vi "Get Directions.vi"(11 "Proto in":refnum<class "Numeric Keypad.lvclass">) -> (2 "Directional Button Presses":string[](array[string]), 3 "Proto out":refnum<class "Numeric Keypad.lvclass">)   [LabVIEW 2020, in "Numeric Keypad.lvclass"]
uses:
  Numeric Keypad.lvclass
  Numeric Keypad.lvclass/Numeric Keypad.ctl
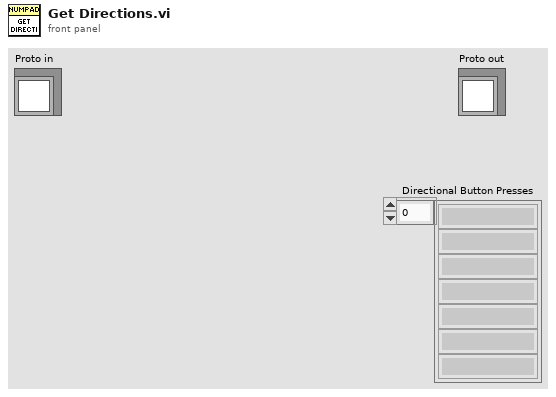
[diagram p1: front panel]
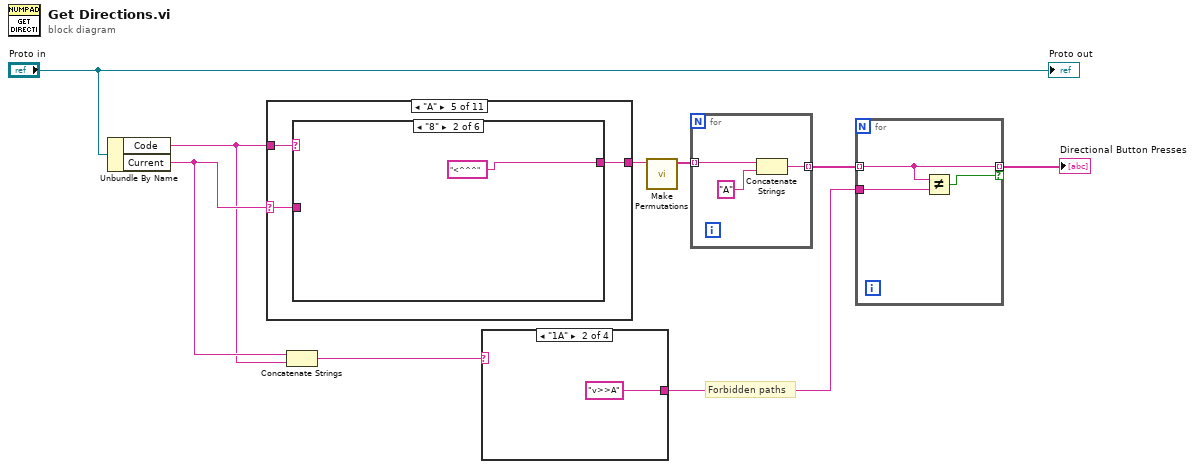
[diagram p0: block diagram]
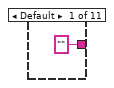
[diagram p2: hidden frame]
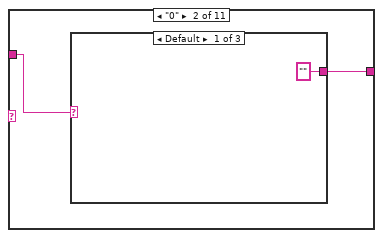
[diagram p3: hidden frame]
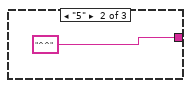
[diagram p4: hidden frame]
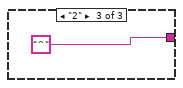
[diagram p5: hidden frame]
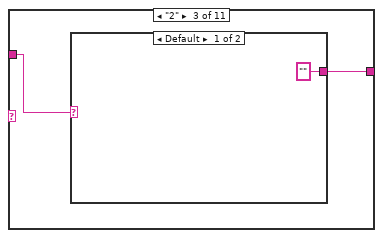
[diagram p6: hidden frame]
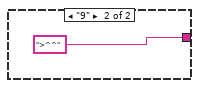
[diagram p7: hidden frame]
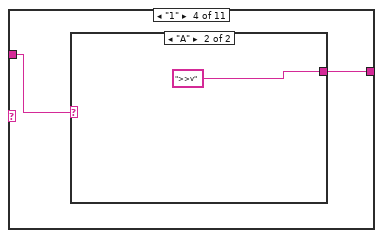
[diagram p8: hidden frame]
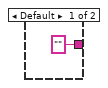
[diagram p9: hidden frame]
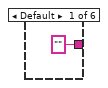
[diagram p10: hidden frame]
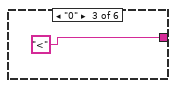
[diagram p11: hidden frame]
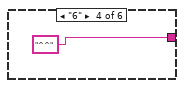
[diagram p12: hidden frame]
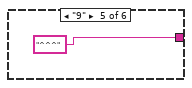
[diagram p13: hidden frame]
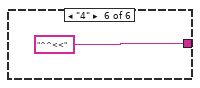
[diagram p14: hidden frame]
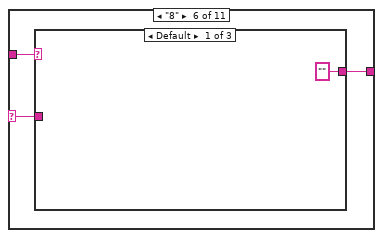
[diagram p15: hidden frame]
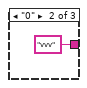
[diagram p16: hidden frame]
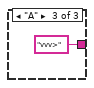
[diagram p17: hidden frame]
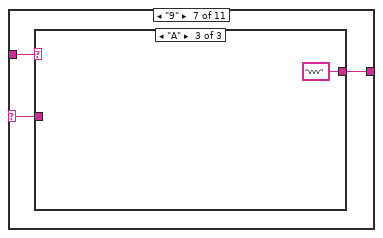
[diagram p18: hidden frame]
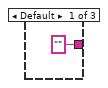
[diagram p19: hidden frame]
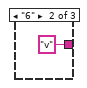
[diagram p20: hidden frame]
diagram:
  # "Forbidden paths"
  n1 = Unbundle By Name("Proto in") -> ("Code"=w5:string, "Current"=w6:string)
  n2 = case shown="\"A\"" w6 {
    selector: w6 -> [_ _ _ _ w25 w34 w40 w46 w52 w58 w65]
    tunnel: w5 -> [_ w11 w16 w20 w26 w35 w41 w47 w53 w59 w66]
    tunnel: ["" w12 w17 w21 w24 w33 w39 w45 w51 w57 w64] -> w8
    frame Default {
    }
    frame "0" {
      n3 = case shown="Default" w11 {
        tunnel: ["" "^^" "^"] -> w12
        frame Default {
        }
        frame "5" {
        }
        frame "2" {
        }
      }
    }
    frame "2" {
      n4 = case shown="Default" w16 {
        tunnel: ["" ">^^"] -> w17
        frame Default {
        }
        frame "9" {
        }
      }
    }
    frame "1" {
      n5 = case shown="\"A\"" w20 {
        tunnel: ["" ">>v"] -> w21
        frame Default {
        }
        frame "A" {
        }
      }
    }
    frame "A" {
      n6 = case shown="\"8\"" w26 {
        tunnel: w25 -> [_ _ _ _ _ _]
        tunnel: ["" "<^^^" "<" "^^" "^^^" "^^<<"] -> w24
        frame Default {
        }
        frame "8" {
        }
        frame "0" {
        }
        frame "6" {
        }
        frame "9" {
        }
        frame "4" {
        }
      }
    }
    frame "8" {
      n7 = case shown="Default" w35 {
        tunnel: w34 -> [_ _ _]
        tunnel: ["" "vvv" "vvv>"] -> w33
        frame Default {
        }
        frame "0" {
        }
        frame "A" {
        }
      }
    }
    frame "9" {
      n8 = case shown="\"A\"" w41 {
        tunnel: w40 -> [_ _ _]
        tunnel: ["" "v" "vvv"] -> w39
        frame Default {
        }
        frame "6" {
        }
        frame "A" {
        }
      }
    }
    frame "5" {
      n9 = case shown="\"9\"" w47 {
        tunnel: w46 -> [_ _ _]
        tunnel: ["" "vv>" ">^"] -> w45
        frame Default {
        }
        frame "A" {
        }
        frame "9" {
        }
      }
    }
    frame "4" {
      n10 = case shown="\"A\"" w53 {
        tunnel: w52 -> [_ _ _]
        tunnel: ["" ">>vv" ">"] -> w51
        frame Default {
        }
        frame "A" {
        }
        frame "5" {
        }
      }
    }
    frame "6" {
      n11 = case shown="\"7\"" w59 {
        tunnel: w58 -> [_ _ _ _]
        tunnel: ["" "<<" "<^" "<<^"] -> w57
        frame Default {
        }
        frame "4" {
        }
        frame "8" {
        }
        frame "7" {
        }
      }
    }
    frame "7" {
      n12 = case shown="\"1\"" w66 {
        tunnel: w65 -> [_ _]
        tunnel: ["" "vv"] -> w64
        frame Default {
        }
        frame "1" {
        }
      }
    }
  }
  n13 = Concatenate Strings(w6, w5) -> (w4:string)
  n14 = case shown="\"1A\"" w4 {
    tunnel: ["" "v>>A" "vv>>A" "<<^^A"] -> w1
    frame Default {
    }
    frame "1A" {
    }
    frame "4A" {
    }
    frame "A4" {
    }
  }
  n15 = call "Make Permutations.vi"("String"=w8) -> ("Array"=w7:string[])  [unwired: 10 in]
  n16 = for {
    tunnel: [w75] -> w2 mode=indexing
    tunnel: w7 -> [w73] mode=indexing
    n17 = Concatenate Strings(w73, "A" ("string")) -> (w75:string)
  }
  n18 = for {
    tunnel: [w78] -> w3 mode=indexing if=w76
    tunnel: w2 -> [w78] mode=indexing
    tunnel: w1 -> [w77]
    n19 = Not Equal?(x=w78, y=w77) -> (x != y?=w76:bool)
  }
  "Directional Button Presses" <- w3
  "Proto out" <- "Proto in"
